vi "SVX9000Basic.vi"() -> ()   [LabVIEW 2011]
uses:
  <vilib>/NI Modbus.llb/MB Ethernet Master Query Write Single Coil (poly).vi
panel:
  out "Output Frequency":sgl
  in  "Device IP Address":string="192.168.1.3"
  in  "Remote Port":u16=502
  in  "Stop App":bool
  in  "Stop VFD":bool
  in  "Start VFD":bool
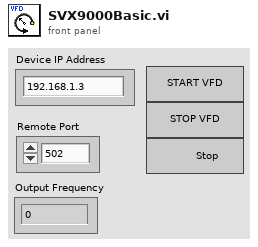
[diagram p1: front panel]
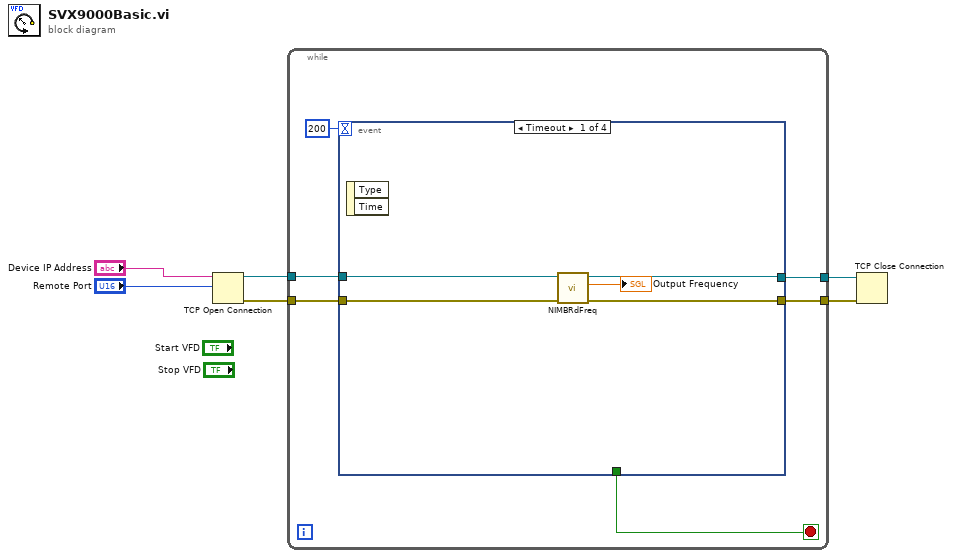
[diagram p0: block diagram]
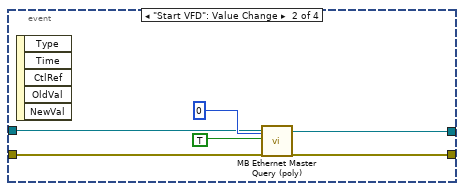
[diagram p2: hidden frame]
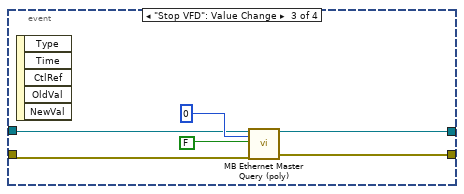
[diagram p3: hidden frame]
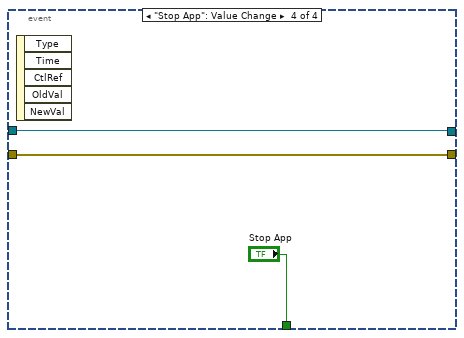
[diagram p4: hidden frame]
diagram:
  n1 = TCP Open Connection(address="Device IP Address", remote port or service name="Remote Port") -> (connection ID=w3:refnum<k5>, error out=w4:errorcluster)  [unwired: 3 in]
  n2 = while {
    tunnel: w4 -> [w12]
    tunnel: w3 -> [w11]
    tunnel: [w9] -> w2
    tunnel: [w8] -> w1
    stop <- w10 stop-if-true
    n3 = event shown="[0] Timeout" {
      selector: _ -> [_ _ _ _]
      dyn-events: _ -> [_ _ _ _]
      timeout: 200 -> [_ _ _ _]
      tunnel: w12 -> [w16 w21 w24 w30]
      tunnel: w11 -> [w17 w20 w28 w31]
      tunnel: [_ _ _ "Stop App"] -> w10
      tunnel: [w15 w19 w26 w31] -> w9
      tunnel: [w14 w18 w25 w30] -> w8
      event Timeout {
        n4 = event-data() -> ()  [unwired: 1 in, 2 out]
        n5 = call "NIMBRdFreq.vi"("error in (no error)"=w16, "TCP Network Connection in"=w17) -> ("error out"=w14:errorcluster, "Output Frequency"=→"Output Frequency":dbl, "TCP Network Connection out"=w15:refnum<k5>)  [unwired: 2 in, 1 out]
      }
      event "Start VFD": Value Change {
        n6 = event-data() -> ()  [unwired: 1 in, 5 out]
        n7 = call-poly <vilib>:"MB Ethernet Master Query (poly).vi"("TCP Connection Refnum in"=w20, "Address"=u16 0, "Coil"=TRUE, "error in"=w21) -> ("TCP Connection Refnum (dup)"=w19:refnum<k5>, "error out"=w18:errorcluster)  [unwired: 13 in, 1 out]
      }
      event "Stop VFD": Value Change {
        n8 = event-data() -> ()  [unwired: 1 in, 5 out]
        n9 = call-poly <vilib>:"MB Ethernet Master Query (poly).vi"("TCP Connection Refnum in"=w28, "Address"=u16 0, "Coil"=FALSE, "error in"=w24) -> ("TCP Connection Refnum (dup)"=w26:refnum<k5>, "error out"=w25:errorcluster)  [unwired: 13 in, 1 out]
      }
      event "Stop App": Value Change {
        n10 = event-data() -> ()  [unwired: 1 in, 5 out]
      }
    }
  }
  n11 = TCP Close Connection(connection ID=w2, error in (no error)=w1) -> ()  [unwired: 1 in, 2 out]
